vi "Enable multiple controls.vi"(9 "Enabled?":bool, 10 "Controls references":refnum<vi>[](array[refnum])) -> ()   [LabVIEW 2011, in "COSYLib.lvlib"]
uses:
  COSYLib.lvlib
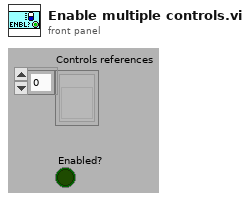
[diagram p1: front panel]
types:
  T1 = enum8{"Enabled", "Disabled", "Disabled and Grayed Out"}
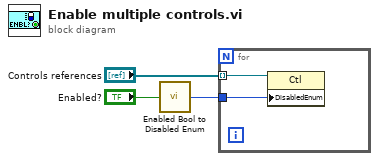
[diagram p0: block diagram]
diagram:
  n1 = call "Enabled Bool to Disabled Enum.vi"("Enabled?"="Enabled?") -> ("Disabled"=w1:T1)
  n2 = for {
    tunnel: "Controls references" -> [w5] mode=indexing
    tunnel: w1 -> [w4]
    n3 = property class="Ctl"(reference=w5, "DisabledEnum"=w4) -> ()  [unwired: 1 in, 2 out]
  }
